vi "Update All Testing with Display.vi"(8 "error in (no error)":errorcluster, 9 "BG Color":u32(colorbox)=16777226, 10 "Message ('')":string, 11 "Application in":refnum<class "Application.lvclass">) -> (0 "error out":errorcluster, 3 "Application out":refnum<class "Application.lvclass">)   [LabVIEW 2017, in "Application.lvlib" / "Application.lvclass"]
doc: "Updates all UUTs in the \"Testing\" state status message with the input \"Message\" and \"BG Color\". Ignores any positions that are not Testing."
uses:
  Application.lvclass
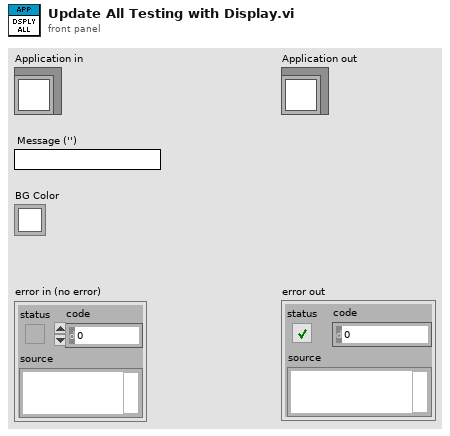
[diagram p1: front panel]
types:
  T1 = cluster{"Serial Number Reference":refnum<vi>, "Status Message Reference":refnum<vi>, "Position":u32}[]
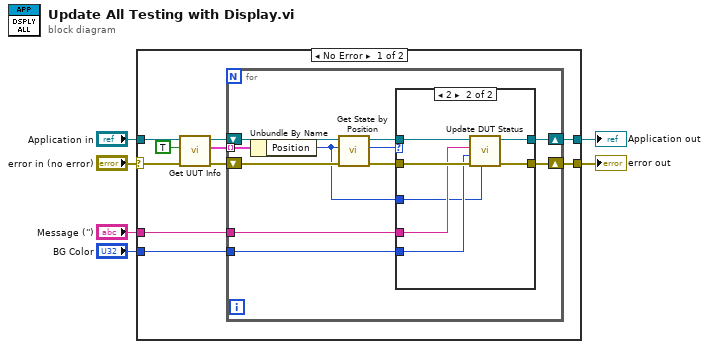
[diagram p0: block diagram]
diagram:
  n1 = case shown="No Error" "error in (no error)" {
    selector: "error in (no error)" -> [w10 w37]
    tunnel: [w16 w38] -> w6
    tunnel: "Application in" -> [w9 w38]
    tunnel: [w15 w37] -> w3
    tunnel: "Message ('')" -> [w14 _]
    tunnel: "BG Color" -> [w13 _]
    frame No Error {
      n2 = call-dynamic "Get UUT Info.vi"("error in (no error)"=w10, "Scanned Only (false)"=TRUE, "Application in"=w9) -> ("error out"=w11:errorcluster, "All UUTs"=w8:T1, "Application out"=w12:refnum<class "Application.lvclass">)  [unwired: 6 in]
      n3 = for {
        shift-right: [w27] -> w16
        shift-left: w12 -> [w25]
        tunnel: w8 -> [w26] mode=indexing
        shift-right: [w21] -> w15
        shift-left: w11 -> [w22]
        tunnel: w14 -> [w18]
        tunnel: w13 -> [w17]
        n4 = Unbundle By Name(w26) -> ("Position"=w19:u32)
        n5 = call-dynamic "Get State by Position.vi"("error in (no error)"=w22, "Position"=w19, "Application in"=w25) -> ("error out"=w20:errorcluster, "State"=w23:u32, "Application out"=w24:refnum<class "Application.lvclass">)  [unwired: 6 in]
        n6 = case shown="2" w23 {
          tunnel: [w29 w36] -> w27
          tunnel: w24 -> [w29 w35]
          tunnel: [w28 w33] -> w21
          tunnel: w20 -> [w28 w34]
          tunnel: w19 -> [_ w30]
          tunnel: w18 -> [_ w32]
          tunnel: w17 -> [_ w31]
          frame 0, Default {
          }
          frame 2 {
            n7 = call "Update DUT Status.vi"("Position"=w30, "error in (no error)"=w34, "BG Color"=w31, "Message ('')"=w32, "Application in"=w35) -> ("error out"=w33:errorcluster, "Application out"=w36:refnum<class "Application.lvclass">)  [unwired: 5 in]
          }
        }
      }
    }
    frame Error {
    }
  }
  "Application out" <- w6
  "error out" <- w3
